vi "ImageDisplayControlDialogBox.vi"(9 "Error Message Out":T1={"Title"="LabVIEW: incorrect VI server settings", "Message"="The current settings of the LabVIEW VI server (Tools Menu>>Options, VI Server: Configuration\nor VI Server: Exported VIs) prevents IMAQ Vision Builder to create the VI.\n\nEnable the Active X protocol and all the server resources,\nand grant access to a VI called \"IVB Create LabVIEW VI.vi\" in the Exported VIs list.", "Buttons"=0, "Icon"=3} {"Icon" items=["No icon", "Stop", "Question", "Exclamation", "Information"]; "Buttons" items=["OK", "OK & Cancel", "Abort, Retry & Ignore", "Yes, No & Cancel", "Yes & No", "Retry & Cancel"]}, 11 "hWnd":u32 format="%.0x") -> (3 "Button pressed":i32(ring) items=["OK", "CANCEL", "ABORT", "RETRY", "IGNORE", "YES", "NO"])   [LabVIEW 2009]
doc: "This VI calls the Windows functions MessageBox and MessageBeep to display a message dialog box and, optionally, play a sound effect. These functions are in the Windows DLL called USER.EXE, which is located in the windows\\system directory. If your computer is not equipped with a sound driver, a short \"beep\" will be played through the PC's speaker.\n\nVarious combinations of dialog boxes are possible. The buttons input selects which buttons are displayed in the dialog box, the icon input determines the icon, if any, and the modality box determines whether the dialog box is system, application, or task modal.\n\nThe following dialog box button schemes are available through the \"buttons\" input:\n0: OK\n1: OK / Cancel\n2: Abort / Retry / Ignore\n3: Yes / No / Cancel\n4: Yes / No\n5: Retry / Cancel\n\nThe following icons are available through the \"icon\" input:\n0: None\n1: STOP icon\n2: Question icon\n3: Exclamation icon\n4: Information icon\n\nThe following three modalities are available:\n0: Application\n1: System\n2: Task\n\nIf sounds are enabled, the icon option determines the sound effect played, as defined in the Sounds section of Windows' Control Panel.\n\nThe DLL functions called are:\n\nint MessageBox ( hWndParent, lpText, lpCaption, wType )\nvoid MessageBeep ( wType )\n\nFunction definitions are from:\nMicrosoft Windows Programmer's Reference\nCopyright 1990 Microsoft Corporation."
uses:
  USER32.DLL
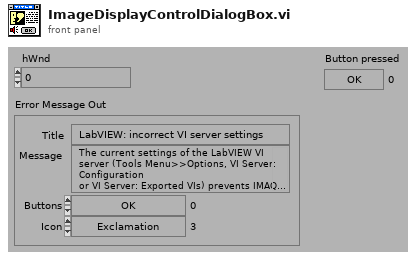
[diagram p1: front panel]
types:
  T1 = cluster{"Title":string, "Message":string, "Buttons":i32, "Icon":i32}
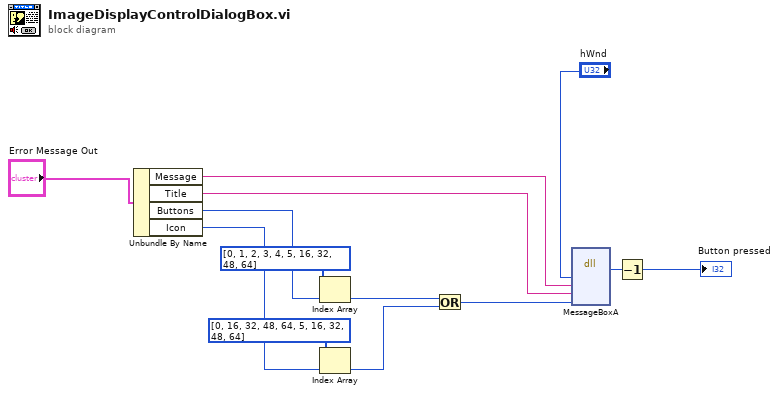
[diagram p0: block diagram]
diagram:
  n1 = Unbundle By Name("Error Message Out") -> ("Message"=w8:string, "Title"=w7:string, "Buttons"=w6:i32, "Icon"=w5:i32)
  n2 = Index Array(array=i32[] [0, 1, 2, 3, 4, 5, 16, 32, 48, 64] ("buttons"), index=w6) -> (element=w12:i32)
  n3 = Index Array(array=i32[] [0, 16, 32, 48, 64, 5, 16, 32, 48, 64] ("icons"), index=w5) -> (element=w11:i32)
  n4 = Or(x=w12, y=w11) -> (x .or. y?=w2:i32)
  n5 = dll-call lib="USER32.DLL" fn="MessageBoxA" label="MessageBox"("hWndParent"="hWnd", "lpText"=w8, "lpCaption"=w7, "wType"=w2) -> (w3:i32)  [unwired: 7 in, 2 out]
  n6 = Decrement(x=w3) -> (x-1=→"Button pressed":i32)
